vi "Initialize.vi"(8 "error in (no error)":errorcluster, 9 "Build Configurations":string[](array[string]), 10 "Preceding Items":refnum<class "Item.lvclass">[](array[class]), 11 "ZIP Item in":refnum<class "ZIP Item.lvclass">) -> (0 "error out":errorcluster, 3 "Item out":refnum<class "Item.lvclass">)   [LabVIEW 2019, in "ZIP.lvlib" / "ZIP Item.lvclass"]
uses:
  ZIP Item.lvclass
  C:/Users/pasca/source/repos/solution-explorer-extensions/libs/Solution.lvlibp/Solution/Item/Item.lvclass
  libs/Solution.lvlibp/Solution/Item/Item.lvclass
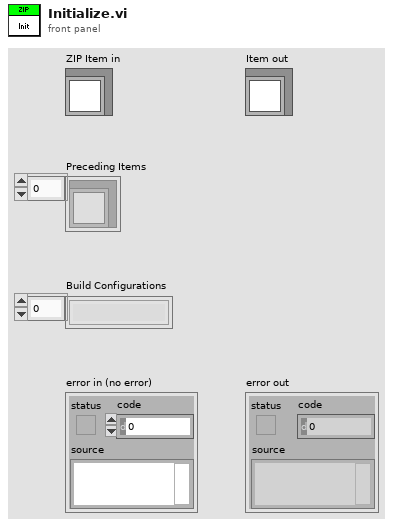
[diagram p1: front panel]
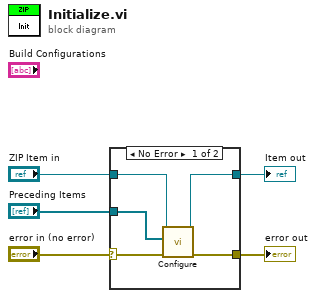
[diagram p0: block diagram]
diagram:
  n1 = case shown="No Error" "error in (no error)" {
    selector: "error in (no error)" -> [w10 w11]
    tunnel: [w9 w11] -> w4
    tunnel: "ZIP Item in" -> [w8 w12]
    tunnel: [w7 w12] -> w2
    tunnel: "Preceding Items" -> [w6 _]
    frame No Error {
      n2 = call "Configure.vi"("error in (no error)"=w10, "Preceding Items"=w6, "ZIP Item in"=w8) -> ("error out"=w9:errorcluster, "ZIP Item out"=w7:refnum<class "ZIP Item.lvclass">)  [unwired: 7 in]
    }
    frame Error {
    }
  }
  "error out" <- w4
  "Item out" <- w2
